vi "Should Stop.vi"(7 "Actor in":refnum<class "Actor.lvclass">, 8 "Error in":errorcluster, 10 "Msg Output":refnum<class "Msg Output.lvclass">) -> (0 "Error out":errorcluster, 2 "Stop":bool, 5 "Actor out":refnum<class "Actor.lvclass">)   [LabVIEW 2020, in "jettl.lvlib"]
uses:
  jettl.lvlib
  Actor/Actor.lvclass
  Msg Output/Msg Output.lvclass
  Msg/Msg.lvclass
  Attributes/Attributes.lvclass
  Transport/Transport.lvclass
  Stop jettl Msg/Stop/Stop.lvlib
  Teardown Location.ctl
  Stop jettl Msg/Stop/Call.vi
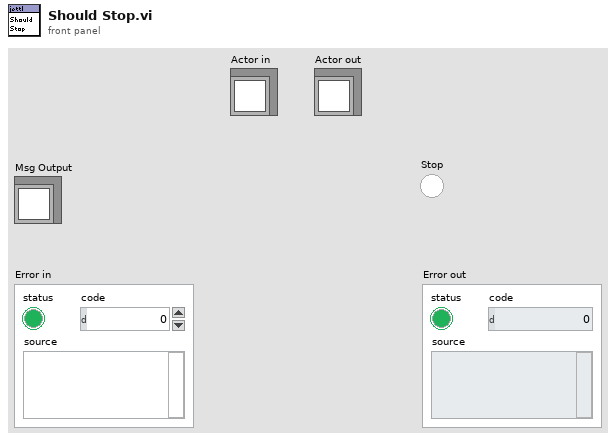
[diagram p1: front panel]
types:
  T1 = typedef "jettl.lvlib/Teardown Location.ctl" = enum16{"Starting", "Should Stop"}
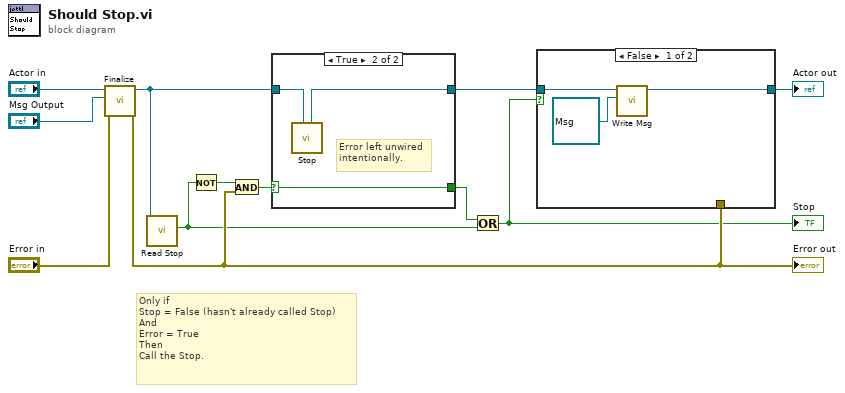
[diagram p0: block diagram]
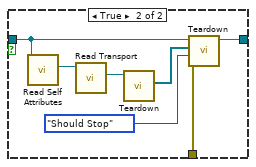
[diagram p3: hidden frame]
diagram:
  # "Only if\nStop = False (hasn't already called Stop)\nAnd\nError = True\nThen\nCall the Stop."
  n1 = call-dynamic "Finalize.vi"("Error in"="Error in", "Msg Output"="Msg Output", "Actor in"="Actor in") -> ("Error out"=w4:errorcluster, "Actor out"=w8:refnum<class "Actor.lvclass">)  [unwired: 7 in]
  "Error out" <- w4
  n2 = call-dynamic "Read Stop.vi"("Actor in"=w8) -> ("Stop"=w3:bool)  [unwired: 10 in]
  n3 = Not(x=w3) -> (.not. x?=w10:bool)
  n4 = And(x=w10, y=w4) -> (x .and. y?=w9:bool)
  n5 = case shown="True" w9 {
    selector: w9 -> [w13 w15]
    tunnel: [w14 w16] -> w7
    tunnel: w8 -> [w14 w17]
    tunnel: [w13 w15] -> w1
    frame False {
    }
    frame True {
      # "Error left unwired intentionally."
      n6 = call-poly "Stop.vi"("Actor in"=w17) -> ("Actor out"=w16:refnum<class "Actor.lvclass">)  [unwired: 9 in, 1 out]
    }
  }
  n7 = Or(x=w1, y=w3) -> (x .or. y?=w2:bool)
  "Stop" <- w2
  n8 = case shown="False" w2 {
    tunnel: w7 -> [w20 w23]
    tunnel: [w19 w22] -> w5
    tunnel: w4 -> [_ w21]
    frame False {
      n9 = call-dynamic "Write Msg.vi"("Msg"=refnum<class "Msg.lvclass"> refnum, "Actor in"=w20) -> ("Actor out"=w19:refnum<class "Actor.lvclass">)  [unwired: 9 in]
    }
    frame True {
      n10 = call-dynamic "Read Self Attributes.vi"("Actor in"=w23) -> ("Self Attributes"=w27:refnum<class "Attributes.lvclass">)  [unwired: 10 in]
      n11 = call-dynamic "Read Transport.vi"("Attributes in"=w27) -> ("Transport"=w26:refnum<class "Transport.lvclass">)  [unwired: 10 in]
      n12 = call-dynamic "Teardown.vi"("Transport in"=w26) -> ("Unheard Msgs"=w25:refnum<class "Msg.lvclass">[])  [unwired: 10 in]
      n13 = call-dynamic "Teardown.vi"("Error in"=w21, "Teardown Location"=Teardown_Location."Should Stop", "Unheard Msgs"=w25, "Actor in"=w23) -> ("Actor out"=w22:refnum<class "Actor.lvclass">)  [unwired: 7 in]
    }
  }
  "Actor out" <- w5
